vi "countEdges.vi"(9 "channel_index":i32=9, 10 "DataPerChannel":dbl[][](array[numeric])=[[5.0, 0.0, 0.0, 5.0, 0.0, 5.0, 0.0, 5.0, 5.0, 5.0, 5.0, 0.0, 0.0], [5.0, 0.0, 0.0, 5.0, 0.0, 5.0, 0.0, 5.0, 0.0, 0.0, 5.0, 0.0, 0.0], [5.0, 0.0, 0.0, 0.0, 5.0, 0.0, 0.0, 5.0, 5.0, 5.0, 5.0, 5.0, 0.0], [5.0, 0.0, 0.0, 0.0, 5.0, 0.0, 0.0, 5.0, 0.0, 0.0, 5.0, 5.0, 0.0], [5.0, 0.0, 0.0, 5.0, 5.0, 5.0, 0.0, 5.0, 0.0, 0.0, 5.0, 5.0, 0.0], [5.0, 0.0, 0.0, 5.0, 5.0, 5.0, 0.0, 5.0, 0.0, 5.0, 5.0, 5.0, 0.0], [5.0, 0.0, 0.0, 5.0, 5.0, 5.0, 0.0, 5.0, 0.0, 0.0, 5.0, 5.0, 0.0], [5.0, 0.0, 0.0, 5.0, 5.0, 5.0, 0.0, 5.0, 0.0, 5.0, 5.0, 5.0, 0.0], [5.0, 0.0, 0.0, 5.0, 5.0, 5.0, 0.0, 5.0, 0.0, 0.0, 5.0, 5.0, 0.0], [5.0, 0.0, 0.0, 5.0, 5.0, 5.0, 0.0, 5.0, 0.0, 5.0, 5.0, 5.0, 0.0], [5.0, 0.0, 0.0, 5.0, 5.0, 5.0, 0.0, 5.0, 0.0, 0.0, 5.0, 5.0, 0.0], [5.0, 0.0, 0.0, 5.0, 5.0, 5.0, 0.0, 5.0, 0.0, 5.0, 5.0, 5.0, 0.0], [5.0, 0.0, 0.0, 5.0, 5.0, 5.0, 0.0, 5.0, 0.0, 0.0, 5.0, 5.0, 0.0], [5.0, 0.0, 0.0, 5.0, 5.0, 5.0, 0.0, 5.0, 0.0, 5.0, 5.0, 5.0, 0.0], [5.0, 0.0, 0.0, 5.0, 5.0, 5.0, 0.0, 5.0, 0.0, 0.0, 5.0, 5.0, 0.0], [5.0, 0.0, 0.0, 5.0, 5.0, 5.0, 0.0, 5.0, 0.0, 5.0, 5.0, 5.0, 0.0], [5.0, 0.0, 0.0, 5.0, 5.0, 5.0, 0.0, 5.0, 0.0, 0.0, 5.0, 5.0, 0.0], [5.0, 0.0, 0.0, 5.0, 5.0, 5.0, 0.0, 5.0, 0.0, 5.0, 5.0, 5.0, 0.0], [5.0, 0.0, 0.0, 5.0, 5.0, 5.0, 0.0, 5.0, 0.0, 0.0, 5.0, 5.0, 0.0], [5.0, 0.0, 0.0, 5.0, 5.0, 5.0, 0.0, 5.0, 0.0, 5.0, 5.0, 5.0, 0.0], [5.0, 0.0, 0.0, 5.0, 5.0, 5.0, 0.0, 5.0, 0.0, 0.0, 5.0, 5.0, 0.0], [5.0, 0.0, 0.0, 5.0, 5.0, 5.0, 0.0, 5.0, 0.0, 5.0, 5.0, 5.0, 0.0], [5.0, 0.0, 0.0, 5.0, 5.0, 5.0, 0.0, 5.0, 0.0, 0.0, 5.0, 5.0, 0.0], [5.0, 0.0, 0.0, 5.0, 5.0, 5.0, 0.0, 5.0, 0.0, 5.0, 5.0, 5.0, 0.0], [5.0, 0.0, 0.0, 5.0, 5.0, 5.0, 0.0, 5.0, 0.0, 0.0, 5.0, 5.0, 0.0], [5.0, 0.0, 0.0, 5.0, 5.0, 5.0, 0.0, 5.0, 0.0, 5.0, 5.0, 5.0, 0.0], [5.0, 0.0, 0.0, 5.0, 5.0, 5.0, 0.0, 5.0, 0.0, 0.0, 5.0, 5.0, 0.0], [5.0, 0.0, 0.0, 5.0, 5.0, 5.0, 0.0, 5.0, 0.0, 5.0, 5.0, 5.0, 0.0], [5.0, 0.0, 0.0, 5.0, 5.0, 5.0, 0.0, 5.0, 0.0, 0.0, 5.0, 5.0, 0.0], [5.0, 0.0, 0.0, 5.0, 5.0, 5.0, 0.0, 5.0, 0.0, 5.0, 5.0, 5.0, 0.0], [5.0, 0.0, 0.0, 5.0, 5.0, 5.0, 0.0, 5.0, 0.0, 0.0, 5.0, 5.0, 0.0], [5.0, 0.0, 0.0, 5.0, 5.0, 5.0, 0.0, 5.0, 0.0, 5.0, 5.0, 5.0, 0.0], [5.0, 0.0, 0.0, 5.0, 5.0, 5.0, 0.0, 5.0, 0.0, 0.0, 5.0, 5.0, 0.0], [5.0, 0.0, 0.0, 5.0, 5.0, 5.0, 0.0, 5.0, 0.0, 5.0, 5.0, 5.0, 0.0], [5.0, 0.0, 0.0, 5.0, 5.0, 5.0, 0.0, 5.0, 0.0, 0.0, 5.0, 5.0, 0.0], [5.0, 0.0, 0.0, 5.0, 5.0, 5.0, 0.0, 5.0, 0.0, 5.0, 5.0, 5.0, 0.0], [5.0, 0.0, 0.0, 5.0, 5.0, 5.0, 0.0, 5.0, 0.0, 0.0, 5.0, 5.0, 0.0], [5.0, 0.0, 0.0, 5.0, 5.0, 5.0, 0.0, 5.0, 0.0, 5.0, 5.0, 5.0, 0.0], [5.0, 0.0, 0.0, 5.0, 5.0, 5.0, 0.0, 5.0, 0.0, 0.0, 5.0, 5.0, 0.0], [5.0, 0.0, 0.0, 5.0, 5.0, 5.0, 0.0, 5.0, 0.0, 5.0, 5.0, 5.0, 0.0], [5.0, 0.0, 0.0, 5.0, 5.0, 5.0, 0.0, 5.0, 0.0, 0.0, 5.0, 5.0, 0.0], [5.0, 0.0, 0.0, 5.0, 5.0, 5.0, 0.0, 5.0, 0.0, 5.0, 5.0, 5.0, 0.0], [5.0, 0.0, 0.0, 5.0, 5.0, 5.0, 0.0, 5.0, 0.0, 0.0, 5.0, 5.0, 0.0], [5.0, 0.0, 0.0, 5.0, 5.0, 5.0, 0.0, 5.0, 0.0, 5.0, 5.0, 5.0, 0.0], [5.0, 0.0, 0.0, 5.0, 5.0, 5.0, 0.0, 5.0, 0.0, 0.0, 5.0, 5.0, 0.0], [5.0, 0.0, 0.0, 5.0, 5.0, 5.0, 0.0, 5.0, 0.0, 5.0, 5.0, 5.0, 0.0], [5.0, 0.0, 0.0, 5.0, 5.0, 5.0, 0.0, 5.0, 0.0, 0.0, 5.0, 5.0, 0.0], [5.0, 0.0, 0.0, 5.0, 5.0, 5.0, 0.0, 5.0, 0.0, 5.0, 5.0, 5.0, 0.0], [5.0, 0.0, 0.0, 5.0, 5.0, 5.0, 0.0, 5.0, 0.0, 0.0, 5.0, 5.0, 0.0], [5.0, 0.0, 0.0, 5.0, 5.0, 5.0, 0.0, 5.0, 0.0, 5.0, 5.0, 5.0, 0.0], [5.0, 0.0, 0.0, 5.0, 5.0, 5.0, 0.0, 5.0, 0.0, 0.0, 5.0, 5.0, 0.0], [5.0, 0.0, 0.0, 5.0, 5.0, 5.0, 0.0, 5.0, 0.0, 5.0, 5.0, 5.0, 0.0], [5.0, 0.0, 0.0, 5.0, 5.0, 5.0, 0.0, 5.0, 0.0, 0.0, 5.0, 5.0, 0.0], [5.0, 0.0, 0.0, 5.0, 5.0, 5.0, 0.0, 5.0, 0.0, 5.0, 5.0, 5.0, 0.0], [5.0, 0.0, 0.0, 5.0, 5.0, 5.0, 0.0, 5.0, 0.0, 0.0, 5.0, 5.0, 0.0], [5.0, 0.0, 0.0, 5.0, 5.0, 5.0, 0.0, 5.0, 0.0, 5.0, 5.0, 5.0, 0.0], [5.0, 0.0, 0.0, 5.0, 5.0, 5.0, 0.0, 5.0, 0.0, 0.0, 5.0, 5.0, 0.0], [5.0, 0.0, 0.0, 5.0, 5.0, 5.0, 0.0, 5.0, 0.0, 5.0, 5.0, 5.0, 0.0], [5.0, 0.0, 0.0, 5.0, 5.0, 5.0, 0.0, 5.0, 0.0, 0.0, 5.0, 5.0, 0.0], [5.0, 0.0, 0.0, 5.0, 5.0, 5.0, 0.0, 5.0, 0.0, 0.0, 5.0, 5.0, 5.0], [5.0, 0.0, 0.0, 5.0, 5.0, 5.0, 0.0, 5.0, 0.0, 0.0, 5.0, 5.0, 0.0], [0.0, 0.0, 5.0, 5.0, 5.0, 5.0, 0.0, 0.0, 0.0, 5.0, 0.0, 5.0, 0.0], [0.0, 0.0, 5.0, 5.0, 5.0, 5.0, 0.0, 0.0, 0.0, 0.0, 0.0, 5.0, 0.0], [0.0, 0.0, 5.0, 5.0, 5.0, 5.0, 0.0, 0.0, 5.0, 0.0, 0.0, 5.0, 0.0], [0.0, 0.0, 5.0, 5.0, 5.0, 5.0, 5.0, 0.0, 0.0, 0.0, 0.0, 5.0, 0.0], [0.0, 0.0, 5.0, 5.0, 5.0, 5.0, 0.0, 0.0, 0.0, 0.0, 0.0, 5.0, 0.0], [0.0, 0.0, 5.0, 5.0, 5.0, 5.0, 5.0, 0.0, 5.0, 0.0, 0.0, 5.0, 0.0], [0.0, 0.0, 5.0, 5.0, 5.0, 5.0, 5.0, 0.0, 0.0, 0.0, 0.0, 5.0, 0.0], [0.0, 0.0, 5.0, 5.0, 5.0, 5.0, 0.0, 0.0, 0.0, 0.0, 0.0, 5.0, 0.0], [0.0, 0.0, 5.0, 5.0, 5.0, 5.0, 0.0, 0.0, 5.0, 0.0, 0.0, 5.0, 0.0], [0.0, 0.0, 5.0, 5.0, 5.0, 5.0, 0.0, 0.0, 0.0, 0.0, 0.0, 5.0, 0.0], [0.0, 0.0, 5.0, 5.0, 5.0, 5.0, 0.0, 0.0, 0.0, 0.0, 0.0, 5.0, 5.0], [0.0, 0.0, 5.0, 5.0, 5.0, 5.0, 0.0, 0.0, 0.0, 0.0, 0.0, 5.0, 0.0], [0.0, 0.0, 5.0, 5.0, 5.0, 5.0, 0.0, 0.0, 0.0, 0.0, 0.0, 5.0, 5.0], [0.0, 0.0, 5.0, 5.0, 5.0, 5.0, 0.0, 0.0, 0.0, 0.0, 0.0, 5.0, 0.0], [0.0, 0.0, 5.0, 5.0, 5.0, 5.0, 5.0, 0.0, 0.0, 0.0, 0.0, 5.0, 0.0], [0.0, 0.0, 5.0, 5.0, 5.0, 5.0, 0.0, 0.0, 0.0, 0.0, 0.0, 5.0, 0.0], [0.0, 0.0, 5.0, 5.0, 5.0, 5.0, 5.0, 0.0, 5.0, 0.0, 0.0, 5.0, 0.0], [0.0, 0.0, 5.0, 5.0, 5.0, 5.0, 5.0, 0.0, 0.0, 0.0, 0.0, 5.0, 0.0], [0.0, 0.0, 5.0, 5.0, 5.0, 5.0, 0.0, 0.0, 0.0, 0.0, 0.0, 5.0, 0.0], [0.0, 0.0, 5.0, 5.0, 5.0, 5.0, 0.0, 0.0, 5.0, 0.0, 0.0, 5.0, 0.0], [0.0, 0.0, 5.0, 5.0, 5.0, 5.0, 0.0, 0.0, 0.0, 0.0, 0.0, 5.0, 0.0], [0.0, 0.0, 5.0, 5.0, 5.0, 5.0, 0.0, 0.0, 0.0, 0.0, 0.0, 5.0, 5.0], [0.0, 0.0, 5.0, 5.0, 5.0, 5.0, 0.0, 0.0, 0.0, 0.0, 0.0, 5.0, 0.0], [0.0, 0.0, 5.0, 5.0, 5.0, 5.0, 0.0, 0.0, 0.0, 5.0, 0.0, 5.0, 0.0], [0.0, 0.0, 5.0, 5.0, 5.0, 5.0, 0.0, 0.0, 0.0, 0.0, 0.0, 5.0, 0.0]]) -> (1 "Number of Changes":i32, 2 "Array":dbl[](array[numeric]))   [LabVIEW 2011, in "run.lvlib"]
uses:
  run.lvlib
  <vilib>/DAQmx/read.llb/DAQmx Read.vi
  <vilib>/DAQmx/read.llb/DAQmx Read (Counter U32 1Chan 1Samp).vi
  <vilib>/DAQmx/create/channels.llb/DAQmx Create Channel (CI-Count Edges).vi
panel:
  out "task out":refnum<k21>
  out "error out":errorcluster
  in  "error in":errorcluster
  in  "stop":bool
  out "data":u32
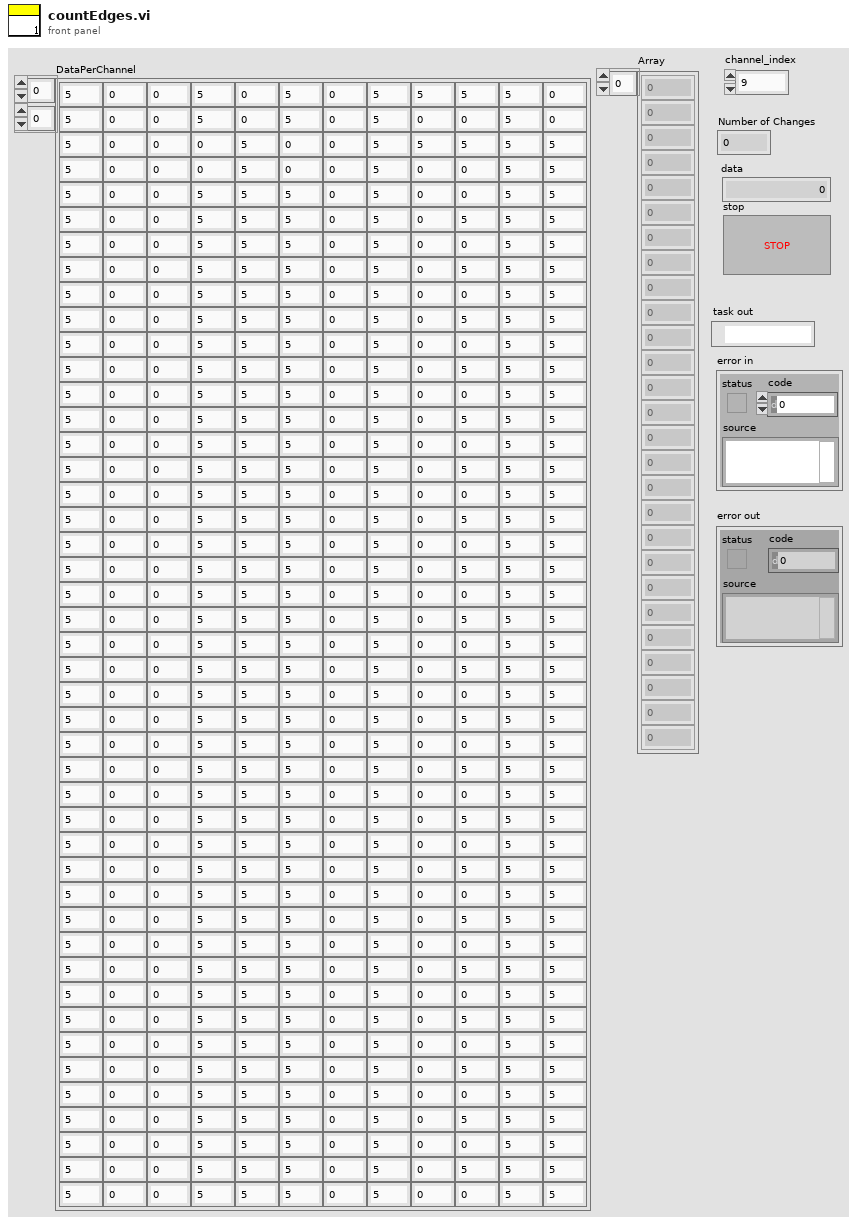
[diagram p1: front panel]
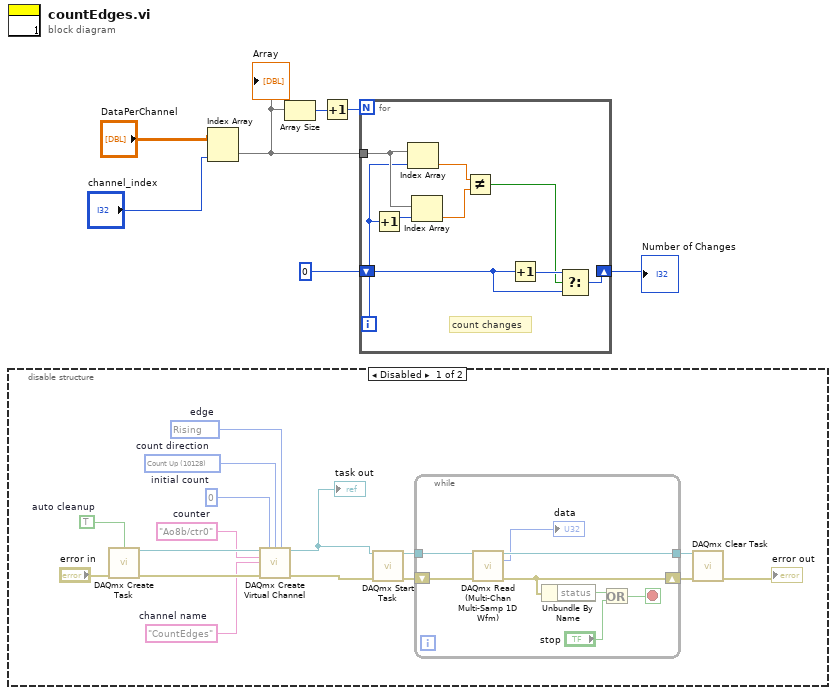
[diagram p0: block diagram]
diagram:
  n1 = disable-structure shown="Disabled" {
    frame Disabled {
      w15 = 10280 items=["Rising"=10280, "Falling"=10171]  # edge
      w16 = 10128 items=["Count Up"=10128, "Count Down"=10124, "Externally Controlled"=10326]  # count direction
      w17 = u32 0  # initial count
      w18 = "CountEdges"  # channel name
      w19 = "Ao8b/ctr0"  # counter
      w21 = TRUE  # auto cleanup
      n2 = call <vilib>:"DAQmx Create Task.vi"("auto cleanup"=w21, "error in"="error in") -> ("task out"=w20:refnum<k21>, "error out"=w22:errorcluster)  [unwired: 3 in, 9 out]
      n3 = call-poly <vilib>:"DAQmx Create Virtual Channel.vi"("task in"=w20, "initial count"=w17, "count direction"=w16, "edge"=w15, "counter"=w19, "name to assign"=w18, "error in"=w22) -> ("task out"=w10:refnum<k21>, "error out"=w9:errorcluster)  [unwired: 7 out]
      "task out" <- w10
      n4 = call <vilib>:"DAQmx Start Task.vi"("task/channels in"=w10, "error in"=w9) -> ("task out"=w14:refnum<k21>, "error out"=w13:errorcluster)  [unwired: 12 out]
      n5 = while {
        tunnel: w14 -> [w31]
        tunnel: [w29] -> w11
        shift-right: [w26] -> w12
        shift-left: w13 -> [w30]
        stop <- w24 stop-if-true
        n6 = call-poly "DAQmx Read (Multi-Chan Multi-Samp 1D Wfm).vi"("task/channels in"=w31, "error in"=w30) -> ("task out"=w29:refnum<k21>, "data"=→"data":u32, "error out"=w26:errorcluster)  [unwired: 1 in, 10 out]
        n7 = Unbundle By Name(w26) -> ("status"=w27:bool)
        n8 = Or(x=w27, y="stop") -> (x .or. y?=w24:bool)
      }
      n9 = call <vilib>:"DAQmx Clear Task.vi"("task in"=w11, "error in"=w12) -> ("error out"=→"error out":errorcluster)  [unwired: 13 out]
    }
    frame Enabled {
    }
  }
  n10 = Index Array(array="DataPerChannel", index (col)="channel_index") -> (element=w3:dbl[])  [unwired: 1 in]
  "Array" <- w3
  n11 = Array Size(array=w3) -> (size(s)=w2:i32)
  n12 = Increment(x=w2) -> (x+1=w1:i32)
  n13 = for {
    N: w1 -> [_]
    tunnel: w3 -> [w40]
    shift-right: [w32] -> w5
    shift-left: 0 -> [w33]
    i -> [w39]
    # "count changes"
    n14 = Increment(x=w39) -> (x+1=w38:i32)
    n15 = Index Array(array=w40, index=w39) -> (element=w36:dbl)
    n16 = Index Array(array=w40, index=w38) -> (element=w37:dbl)
    n17 = Not Equal?(x=w36, y=w37) -> (x != y?=w34:bool)
    n18 = Increment(x=w33) -> (x+1=w35:i32)
    n19 = Select(t=w35, s=w34, f=w33) -> (s? t:f=w32:i32)
  }
  "Number of Changes" <- w5
